vi "Launch Asynchronous Execution Units.vi"(8 "error in (no error)":errorcluster, 10 "RTStateVariables in":T2 {"Inline Execution Units"."Outgoing Data References"."Data Reference" format="%.0x"; "Inline Execution Units"."Incoming Data References" format="%.0x"}, 11 "Device Ref in":T1 format="%.0x") -> (0 "error out":errorcluster, 2 "RTStateVariables out":T2 {"Inline Execution Units"."Outgoing Data References"."Data Reference" format="%.0x"; "Inline Execution Units"."Incoming Data References" format="%.0x"}, 3 "Device Ref out":T1 format="%.0x")   [LabVIEW 2023, in "Ballard MIL-STD-1553 Engine Support.lvlib" / "Custom Device.lvlib"]
uses:
  Custom Device.lvlib
  RTStateVariables.ctl
  <vilib>/NI/NIVS Inline Async API/_VS Inline Async API/VS Inline Async API/VS Inline Async API.lvclass
  Interfaces/Shared Resources/Shared Resources.lvclass
  Inline Execution Unit Runtime Information.ctl
  Interfaces/Execution Unit/Execution Unit.lvclass
  <vilib>/NI VeriStand/Custom Device API/Data Reference.ctl
  <vilib>/NI VeriStand/Custom Device API/Block Data Reference.ctl
  Asynchronous Execution Unit Runtime Information.ctl
  <vilib>/NI VeriStand/Custom Device API/Custom Device Item Ref.ctl
  Asynchronous Process Parameters.ctl
  Execution Unit.Async.vi
  <vilib>/NI VeriStand/Custom Device Tools/Custom Device Utility Library/Custom Device Utility Library.lvlib
  <vilib>/NI VeriStand/Custom Device API/Custom Device API.lvlib
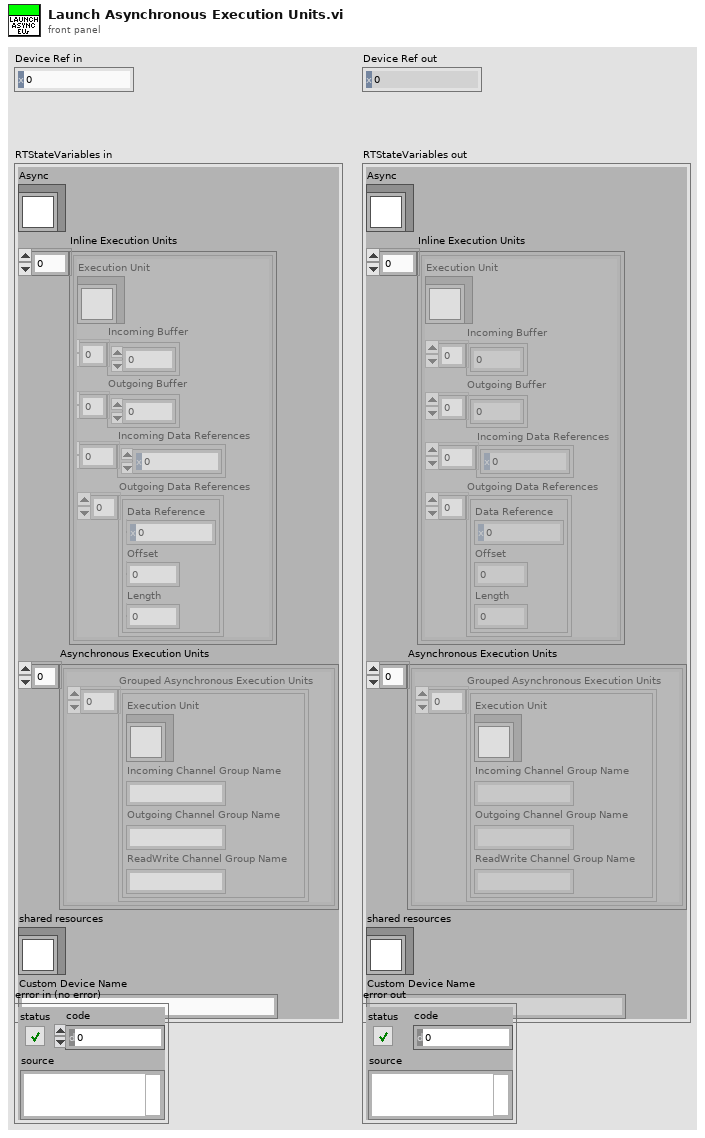
[diagram p1: front panel]
types:
  T1 = typedef "Custom Device API.lvlib/Custom Device Item Ref.ctl" = u64
  T2 = typedef "Ballard MIL-STD-1553 Engine Support.lvlib/Custom Device.lvlib/RTStateVariables.ctl" = cluster{"Async":refnum<class "VS Inline Async API.lvclass">, "Inline Execution Units":T3[], "Asynchronous Execution Units":cluster{"Grouped Asynchronous Execution Units":T6[]}[], "shared resources":refnum<class "Shared Resources.lvclass">, "Custom Device Name":string}
  T3 = typedef "Ballard MIL-STD-1553 Engine Support.lvlib/Custom Device.lvlib/Inline Execution Unit Runtime Information.ctl" = cluster{"Execution Unit":refnum<class "Execution Unit.lvclass">, "Incoming Buffer":dbl[], "Outgoing Buffer":dbl[], "Incoming Data References":T4[], "Outgoing Data References":T5[]}
  T4 = typedef "Custom Device API.lvlib/Data Reference.ctl" = i32
  T5 = typedef "Custom Device API.lvlib/Block Data Reference.ctl" = cluster{"Data Reference":T4, "Offset":u64, "Length":u64}
  T6 = typedef "Ballard MIL-STD-1553 Engine Support.lvlib/Custom Device.lvlib/Asynchronous Execution Unit Runtime Information.ctl" = cluster{"Execution Unit":refnum<class "Execution Unit.lvclass">, "Incoming Channel Group Name":string, "Outgoing Channel Group Name":string, "ReadWrite Channel Group Name":string}
  T7 = cluster{"Grouped Asynchronous Execution Units":T6[]}[]
  T8 = typedef "Ballard MIL-STD-1553 Engine Support.lvlib/Custom Device.lvlib/Asynchronous Process Parameters.ctl" = cluster{"Grouped Asynchronous Execution Unit Runtime Information":T6[], "shared resources":refnum<class "Shared Resources.lvclass">}
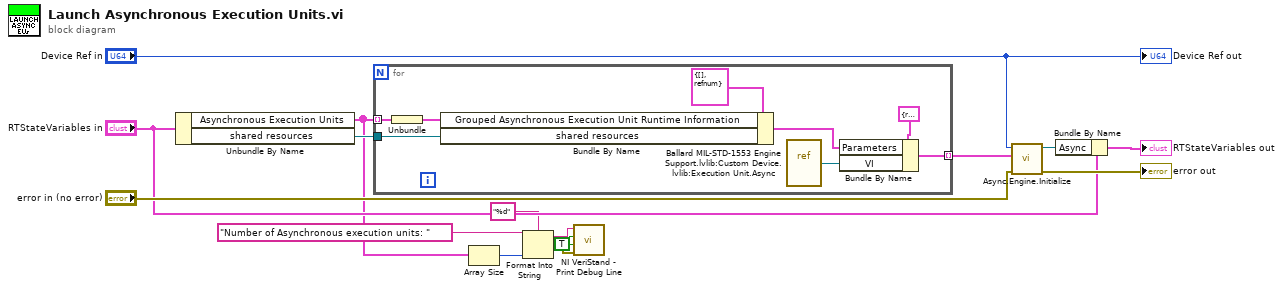
[diagram p0: block diagram]
diagram:
  w2 = TRUE ("Append newline? (T)")
  n1 = Unbundle By Name("RTStateVariables in") -> ("Asynchronous Execution Units"=w1:T7, "shared resources"=w8:refnum<class "Shared Resources.lvclass">)
  n2 = for {
    tunnel: w1 -> [w19] mode=indexing
    tunnel: [w22] -> w9 mode=indexing
    tunnel: w8 -> [w18]
    n3 = Unbundle(w19) -> ("Grouped Asynchronous Execution Units"=w16:T6[])
    n4 = Bundle By Name(cluster=T8 {"Grouped Asynchronous Execution Unit Runtime Information"=[], "shared resources"=refnum} ("Asynchronous Process Parameters"), "Grouped Asynchronous Execution Unit Runtime Information"=w16, "shared resources"=w18) -> (w17:T8)
    n5 = vi-ref "Ballard MIL-STD-1553 Engine Support.lvlib:Custom Device.lvlib:Execution Unit.Async.vi"() -> (w21:refnum<vi>)
    n6 = Bundle By Name(cluster=cluster{"VI":refnum<vi>, "Parameters":variant} {"VI"=refnum, "Parameters"=variant} ("Process"), "Parameters"=w17, "VI"=w21) -> (w22:cluster{"VI":refnum<vi>, "Parameters":variant})
  }
  n7 = Array Size(array=w1) -> (size(s)=w6:i32)
  n8 = Format Into String(format string="%d", initial string="Number of Asynchronous execution units: ", w6) -> (resulting string=w3:string, error out=w7:errorcluster)  [unwired: 1 in]
  n9 = call <vilib>:"NI VeriStand - Print Debug Line.vi"("error in (no error)"=w7, "Append newline? (T)"=w2, "Add to log file? (F)"=w2, "Message"=w3) -> ()  [unwired: 7 in, 1 out]
  n10 = call <vilib>:"Async.Engine.Initialize.vi"("error in (no error)"="error in (no error)", "Processes"=w9, "Custom Device Ref"="Device Ref in") -> ("error out"=→"error out":errorcluster, "Async"=w11:refnum<class "VS Inline Async API.lvclass">)  [unwired: 7 in]
  n11 = Bundle By Name(cluster="RTStateVariables in", "Async"=w11) -> (→"RTStateVariables out":T2)
  "Device Ref out" <- "Device Ref in"
